vi "main_program.vi"   [LabVIEW 2014]
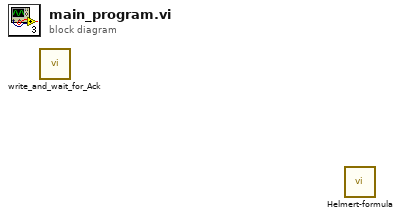
[diagram p0: block diagram]
diagram:
  n1 = call "write_and_wait_for_Ack.vi"() -> ()  [unwired: 7 in, 3 out]
  n2 = call "Helmert-formula.vi"() -> ()  [unwired: 8 in, 4 out]
